vi "Initialize.vi"(7 "Serial Configuration":T1={"Baud Rate"=9600, "Parity"=0, "Data Bits"=7, "Stop Bits"=10, "Flow Control"=0} {"Flow Control" items=["None", "XON/XOFF", "RTS/CTS", "XON/XOFF & RTS/CTS", "DTR/DSR", "XON/XOFF & DTR/DSR"]; "Stop Bits" items=["1.0"=10, "1.5"=15, "2.0"=20]; "Data Bits" items=["7"=7, "8"=8]; "Parity" items=["None", "Odd", "Even", "Mark", "Space"]; "Baud Rate" items=["300"=300, "600"=600, "1200"=1200, "2400"=2400, "4800"=4800, "9600"=9600, "19200"=19200]}, 8 "error in (no error)":errorcluster, 9 "Reset (True)":bool=TRUE, 10 "ID Query (True)":bool=TRUE, 11 "VISA resource name":refnum<visa-resource-name>) -> (0 "error out":errorcluster, 3 "VISA resource name out":refnum<visa-resource-name>)   [LabVIEW 2018, in "Keithley 622X.lvlib"]
doc: "Establishes communication with the instrument and optionally performs an instrument identification query and/or an instrument reset. It also places the instrument in a default state needed for other instrument driver operations. Therefore, call this VI before calling other instrument driver VIs for this instrument. Generally, you need to call the Initialize VI only once at the beginning of an application."
uses:
  <instrlib>/Keithley 622x/Keithley 622X.lvlib
panel:
  # "(c) 2008 Keithley Instruments Inc.  ALL RIGHTS RESERVED."
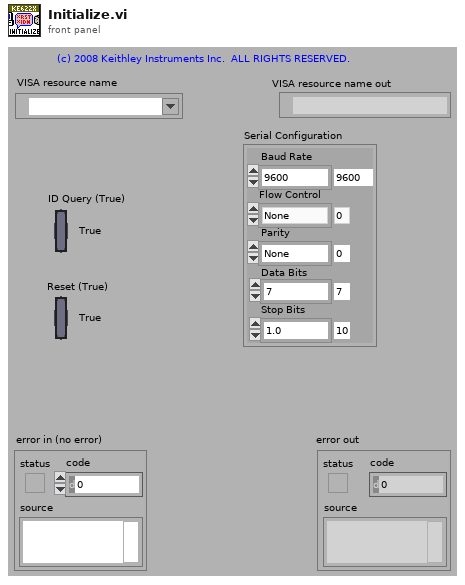
[diagram p1: front panel]
types:
  T1 = cluster{"Baud Rate":u32, "Parity":u16, "Data Bits":u16, "Stop Bits":u16, "Flow Control":u16}
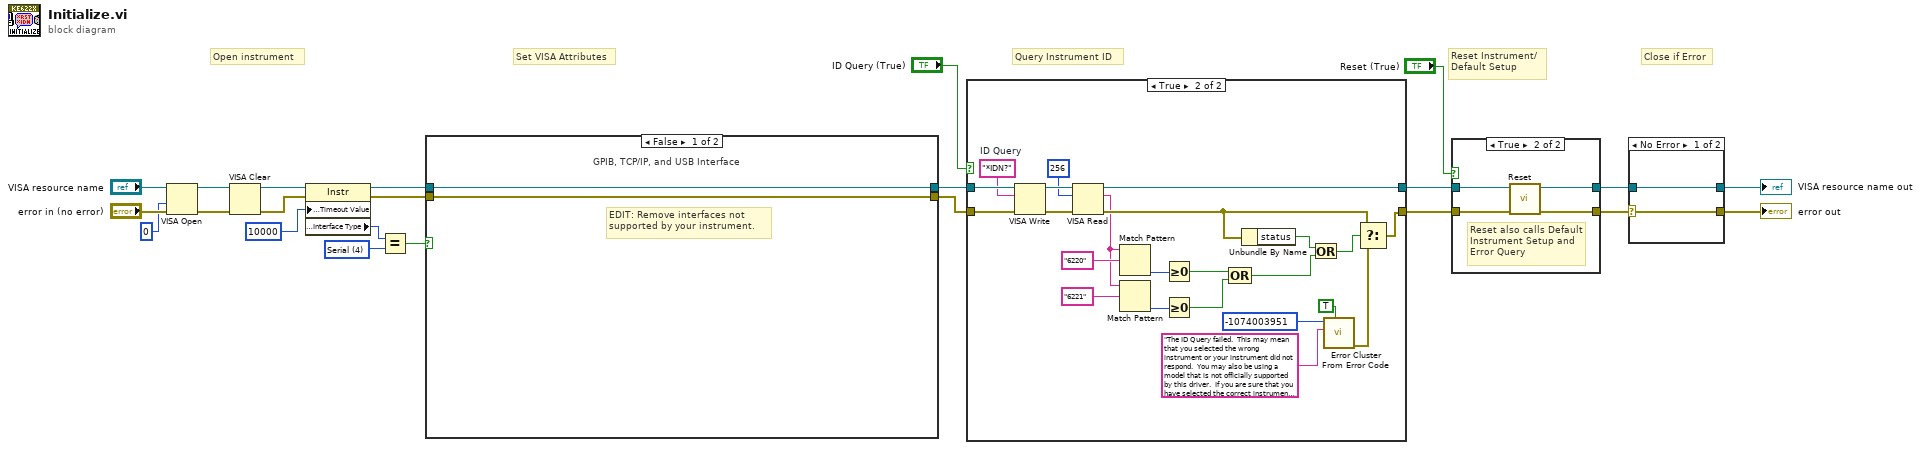
[diagram p0: block diagram]
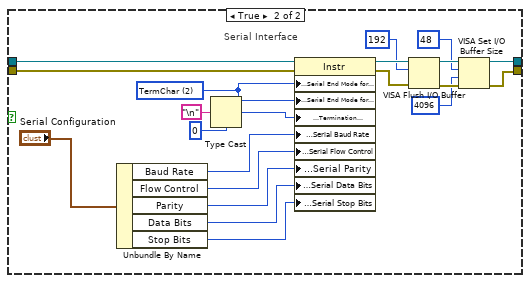
[diagram p2: hidden frame]
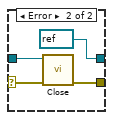
[diagram p3: hidden frame]
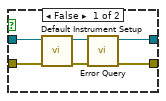
[diagram p4: hidden frame]
diagram:
  w10 = u16 4 items=["GPIB"=1, "VXI"=2, "GPIB-VXI"=3, "Serial"=4, "PXI"=5, "TCPIP"=6, "USB"=7] ("Interface Information:Interface Type")
  # "Set VISA Attributes"
  # "Close if Error"
  # "Query Instrument ID"
  # "Reset Instrument/\nDefault Setup"
  # "Open instrument"
  n1 = VISA Open(access mode=u32 0, error in (no error)="error in (no error)", VISA resource name="VISA resource name") -> (VISA resource name=w8:refnum<visa-resource-name>, error out=w7:errorcluster)  [unwired: 2 in]
  n2 = VISA Clear(VISA resource name=w8, error in (no error)=w7) -> (VISA resource name out=w6:refnum<visa-resource-name>, error out=w5:errorcluster)
  n3 = property class="Instr"(reference=w6, error in=w5, "General Settings:Timeout Value"=u32 10000) -> (reference out=w13:refnum<visa-resource-name>, error out=w12:errorcluster, "Interface Information:Interface Type"=w17:u16)
  n4 = Equal?(x=w17, y=w10) -> (x = y?=w11:bool)
  n5 = case shown="False" w11 {
    tunnel: [w24 w43] -> w15
    tunnel: [w25 w40] -> w14
    tunnel: w13 -> [w24 w45]
    tunnel: w12 -> [w25 w46]
    frame False {
      # "EDIT: Remove interfaces not\nsupported by your instrument."
      # "GPIB, TCP/IP, and USB Interface"
    }
    frame True {
      w33 = u16 2 items=["None", "LastBit", "TermChar"] ("Serial Settings:Serial End Mode for Reads")
      # "Serial Interface"
      n6 = Unbundle By Name("Serial Configuration") -> ("Baud Rate"=w31:u32, "Flow Control"=w27:u16, "Parity"=w29:u16, "Data Bits"=w30:u16, "Stop Bits"=w26:u16)
      n7 = Type Cast(type=u8 0, x="\n" ("Line Feed Constant")) -> (*(type *) &x=w32:u8)
      n8 = property class="Instr"(reference=w45, error in=w46, "Serial Settings:Serial End Mode for Reads"=w33, "Serial Settings:Serial End Mode for Writes"=w33, "Message Based Settings:Termination Character"=w32, "Serial Settings:Serial Baud Rate"=w31, "Serial Settings:Serial Flow Control"=w27, "Serial Settings:Serial Parity"=w29, "Serial Settings:Serial Data Bits"=w30, "Serial Settings:Serial Stop Bits"=w26) -> (reference out=w39:refnum<visa-resource-name>, error out=w42:errorcluster)
      n9 = VISA Flush I/O Buffer(VISA resource name=w39, mask (16)=u16 192, error in (no error)=w42) -> (VISA resource name out=w44:refnum<visa-resource-name>, error out=w41:errorcluster)
      n10 = VISA Set I/O Buffer Size(VISA resource name=w44, mask (16)=u16 48, size (4096)=u32 4096 ("size (0)"), error in (no error)=w41) -> (VISA resource name out=w43:refnum<visa-resource-name>, error out=w40:errorcluster)
    }
  }
  n11 = case shown="True" "ID Query (True)" {
    tunnel: [w47 w71] -> w22
    tunnel: [w48 w68] -> w23
    tunnel: w15 -> [w48 w69]
    tunnel: w14 -> [w47 w70]
    frame False {
    }
    frame True {
      w63 = "*IDN?"  # ID Query
      n12 = VISA Write(VISA resource name=w69, write buffer=w63, error in (no error)=w70) -> (VISA resource name out=w67:refnum<visa-resource-name>, error out=w66:errorcluster)  [unwired: 1 out]
      n13 = VISA Read(VISA resource name=w67, byte count=u32 256, error in (no error)=w66) -> (VISA resource name out=w68:refnum<visa-resource-name>, read buffer=w49:string, error out=w57:errorcluster)  [unwired: 1 out]
      n14 = Match Pattern(string=w49, regular expression="6220") -> (offset past match=w58:i32)  [unwired: 1 in, 3 out]
      n15 = Match Pattern(string=w49, regular expression="6221") -> (offset past match=w54:i32)  [unwired: 1 in, 3 out]
      n16 = Greater Or Equal To 0?(x=w58) -> (x >= 0?=w51:bool)
      n17 = Greater Or Equal To 0?(x=w54) -> (x >= 0?=w52:bool)
      n18 = Compound Arithmetic op=OR(w51, w52) -> (w50:bool)
      n19 = Unbundle By Name(w57) -> ("status"=w56:bool)
      n20 = Or(x=w56, y=w50) -> (x .or. y?=w55:bool)
      n21 = call <vilib>:"Error Cluster From Error Code.vi"("show call chain? (False)"=TRUE, "error message (\"\")"="The ID Query failed.  This may mean that you selected the wrong instrument or your instrument did not respond.  You may also be using a model that is not officially supported by this driver.  If you are sure that you have selected the correct instrument and it is responding, try disabling the ID Query." ("Source (VI Name)"), "error code (0)"=-1074003951 ("Code")) -> ("error out"=w62:errorcluster)  [unwired: 6 in]
      n22 = Select(t=w57, s=w55, f=w62) -> (s? t:f=w71:errorcluster)
    }
  }
  n23 = case shown="True" "Reset (True)" {
    tunnel: w22 -> [w76 w78]
    tunnel: [w73 w81] -> w1
    tunnel: w23 -> [w77 w79]
    tunnel: [w74 w80] -> w2
    frame False {
      n24 = call <instrlib>:"Default Instrument Setup.vi"("error in (no error)"=w76, "VISA resource name"=w77) -> ("error out"=w72:errorcluster, "VISA resource name out"=w75:refnum<visa-resource-name>)  [unwired: 8 in]
      n25 = call <instrlib>:"Error Query.vi"("error in (no error)"=w72, "VISA resource name"=w75) -> ("error out"=w73:errorcluster, "VISA resource name out"=w74:refnum<visa-resource-name>)  [unwired: 6 in, 2 out]
    }
    frame True {
      # "Reset also calls Default Instrument Setup and Error Query"
      n26 = call <instrlib>:"Reset.vi"("error in (no error)"=w78, "VISA resource name"=w79) -> ("error out"=w81:errorcluster, "VISA resource name out"=w80:refnum<visa-resource-name>)  [unwired: 8 in]
    }
  }
  n27 = case shown="No Error" w1 {
    selector: w1 -> [w82 w85]
    tunnel: w2 -> [w83 w86]
    tunnel: [w83 refnum<visa-resource-name> refnum ("VISA resource name out")] -> w4
    tunnel: [w82 w87] -> w3
    frame No Error {
    }
    frame Error {
      n28 = call <instrlib>:"Close.vi"("error in (no error)"=w85, "VISA resource name"=w86) -> ("error out"=w87:errorcluster)  [unwired: 9 in]
    }
  }
  "VISA resource name out" <- w4
  "error out" <- w3
